vi "Chemical Oxidizer.vi"(7 "Speed Upgrades":u32 max=8, 10 "Items/t In":ext, 11 "Input":u16(ring) items=["Sulfur Dust", "Yellow Cake Uranium", "Yellow Cake Uranium Block"]) -> (1 "Input Limiting":bool, 2 "Limiting":bool, 3 "Output Gas (mB/t)":ext format="%.2f", 4 "Required Items/t":ext, 6 "Required Items/s":ext)   [LabVIEW 2023]
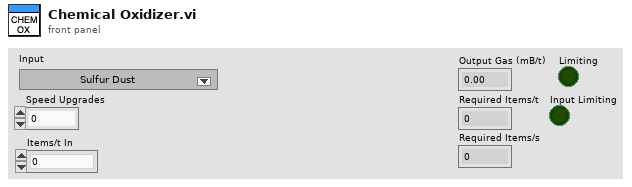
[diagram p1: front panel]
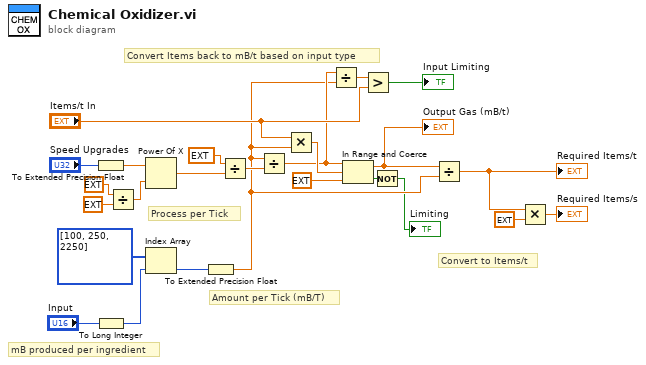
[diagram p0: block diagram]
diagram:
  # "Convert to Items/t"
  # "mB produced per ingredient"
  # "Convert Items back to mB/t based on input type"
  # "Amount per Tick (mB/T)"
  # "Process per Tick"
  n1 = To Extended Precision Float(1:"Speed Upgrades") -> (0:w17:ext)
  n2 = To Long Integer(number="Input") -> (32bit integer=w14:i32)
  n3 = Divide(x=ext 4.0, y=ext 3.0) -> (x/y=w19:ext)
  n4 = Power Of X(1:w19, 2:w17) -> (0:w23:ext)
  n5 = Index Array(array=i32[] [100, 250, 2250], index=w14) -> (element=w13:i32)
  n6 = To Extended Precision Float(1:w13) -> (0:w2:ext)
  n7 = Divide(x=ext 100.0 ("y"), y=w23) -> (x/y=w24:ext)
  n8 = Divide(x=w2, y=w24) -> (x/y=w4:ext)
  n9 = Multiply(x="Items/t In", y=w2) -> (x*y=w6:ext)
  n10 = Divide(x=w4, y=w2) -> (x/y=w3:ext)
  n11 = In Range and Coerce(upper limit=w4, x=w6, lower limit=ext 0.0) -> (coerced(x)=w8:ext, In Range?=w5:bool)
  "Output Gas (mB/t)" <- w8
  n12 = Greater?(x=w3, y="Items/t In") -> (0:→"Input Limiting":bool)
  n13 = Not(x=w5) -> (.not. x?=→"Limiting":bool)
  n14 = Divide(x=w8, y=w2) -> (x/y=w10:ext)
  "Required Items/t" <- w10
  n15 = Multiply(x=w10, y=ext 20.0) -> (x*y=→"Required Items/s":ext)
